vi "Clousure.vi"(8 "error in (no error)":errorcluster, 11 "CreatorB":refnum<class "CreatorB.lvclass">) -> (0 "error out":errorcluster, 3 "CreatorB":refnum<class "CreatorB.lvclass">)   [LabVIEW 2020, in "FactoryMethod.lvlib" / "FactoryMethodLazyEvaluation.lvlib" / "CreatorB.lvclass"]
uses:
  CreatorB.lvclass
  Creator/Creator.lvclass
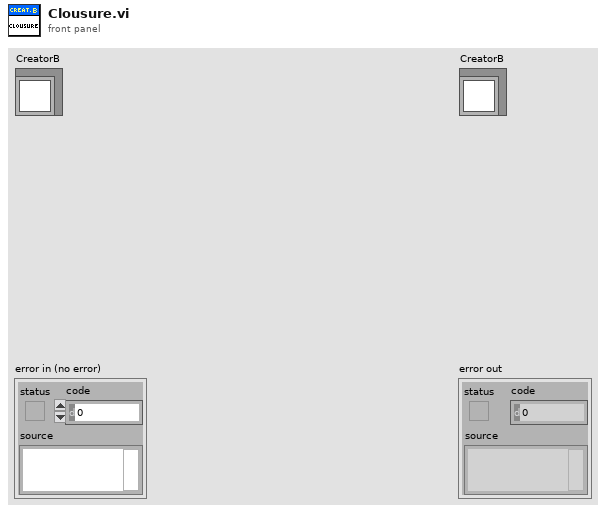
[diagram p1: front panel]
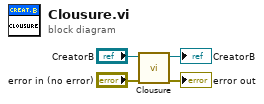
[diagram p0: block diagram]
diagram:
  n1 = call-parent "Clousure.vi"("error in (no error)"="error in (no error)", "Creator in"="CreatorB") -> ("error out"=→"error out":errorcluster, "Creator out"=→"CreatorB":refnum<class "CreatorB.lvclass">)  [unwired: 8 in]
